vi "Read settings node (as text).vi"(8 "error in (no error)":errorcluster, 9 "Create if necessary? (FALSE)":bool, 10 "Settings node name":string, 11 "CoSy Config File in":refnum<class "CoSy Config File.lvclass">) -> (0 "error out":errorcluster, 1 "Created?":bool, 2 "Settings node contents":string, 3 "CoSy Config File out":refnum<class "CoSy Config File.lvclass">)   [LabVIEW 2011, in "COSYLib.lvlib" / "CoSy Config File.lvclass"]
doc: "Retrieve the contents of a <B>settings node</B> (a node directly under the root node) as an XML string.\nIf <B>Create if necessary?</B> is TRUE, the settings node will be created automatically if it doesn't exist yet."
uses:
  CoSy Config File.lvclass
  <vilib>/xml/Close Reference(Node).vi
  <vilib>/xml/NI_XML.lvlib
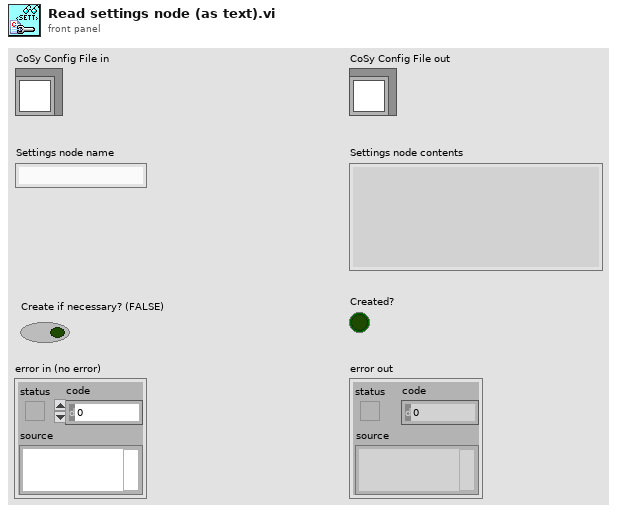
[diagram p1: front panel]
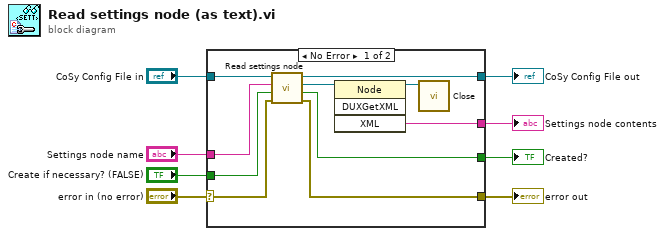
[diagram p0: block diagram]
diagram:
  n1 = case shown="No Error" "error in (no error)" {
    selector: "error in (no error)" -> [w14 w20]
    tunnel: [w9 w20] -> w7
    tunnel: [w17 w19] -> w5
    tunnel: "CoSy Config File in" -> [w18 w19]
    tunnel: "Settings node name" -> [w16 _]
    tunnel: "Create if necessary? (FALSE)" -> [w15 _]
    tunnel: [w12 _] -> w2
    tunnel: [w10 _] -> w1
    frame No Error {
      n2 = call "Read settings node.vi"("error in (no error)"=w14, "Create if necessary? (FALSE)"=w15, "Settings node name"=w16, "CoSy Config File in"=w18) -> ("error out"=w9:errorcluster, "Created?"=w10:bool, "Settings node"=w13:refnum<k20>, "CoSy Config File out"=w17:refnum<class "CoSy Config File.lvclass">)  [unwired: 4 in]
      n3 = invoke class="Node" method="DUXGetXML"(reference=w13) -> (reference out=w11:refnum<k20>, "XML"=w12:string)  [unwired: 3 in, 2 out]
      n4 = call-poly <vilib>:"Close.vi"("node"=w11) -> ()  [unwired: 8 in, 1 out]
    }
    frame Error {
    }
  }
  "error out" <- w7
  "CoSy Config File out" <- w5
  "Created?" <- w1
  "Settings node contents" <- w2
